vi "FTP上传UI.vi"() -> ()   [LabVIEW 2016]
uses:
  <vilib>/FTP/NI_FTP.lvlib
panel:
  out "大小（字节）":i64
  out "remote path":string
  out "temp path":path
  in  "上传版本txt":bool
  in  "read txt":bool
  in  "更新版本记录txt":string
  out "上传中":bool
  in  "remote port (21)":u16=21 caption="远程端口(21)"
  in  "password":string="std23506" caption="密码"
  in  "user":string="update" caption="用户"
  in  "host":string="27.154.58.30" caption="主机"
  in  "transfer spec":cluster{"remote path":string, "local path":path}={"remote path"="数据传输系统\\平台数据传输系统.exe\r\n", "local path"=path "C:/LabVIEW Project/builds/NEW平台数据传输系统/平台数据传输系统.exe"} caption="传输规范"
  in  "上传程序":bool
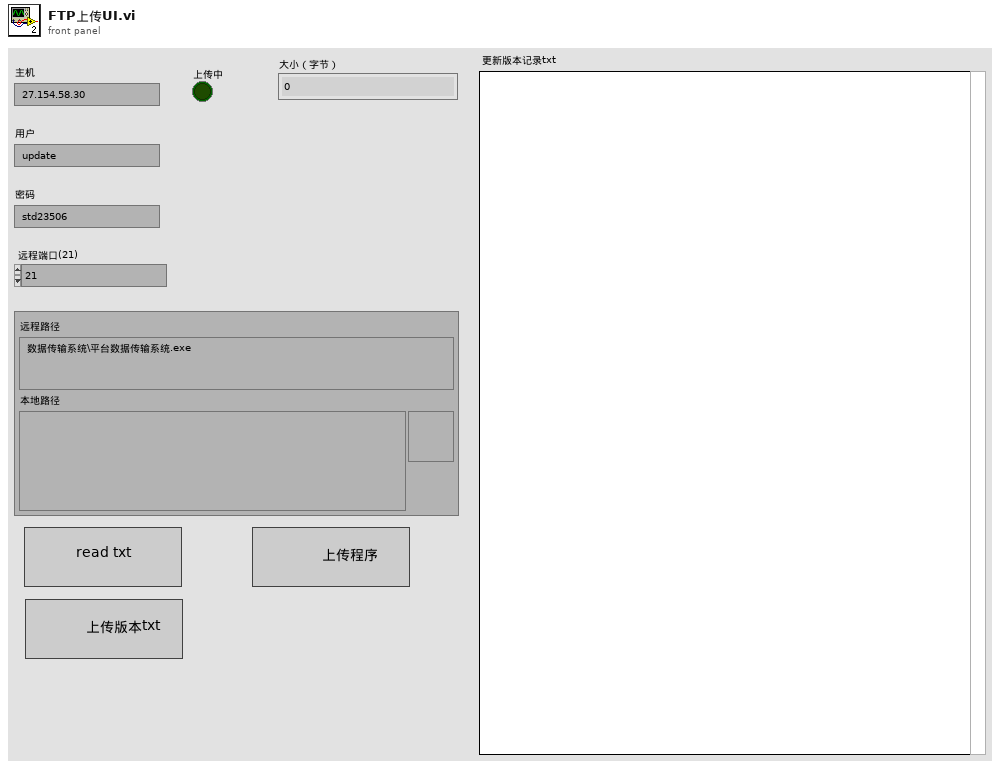
[diagram p1: front panel]
types:
  T1 = enum8{"Enabled", "Disabled", "Disabled and Grayed Out"}
  T2 = cluster{"remote path":string, "local path":path, "binary":bool}
  T3 = cluster{"remote path":string, "local path":path, "binary":bool}[]
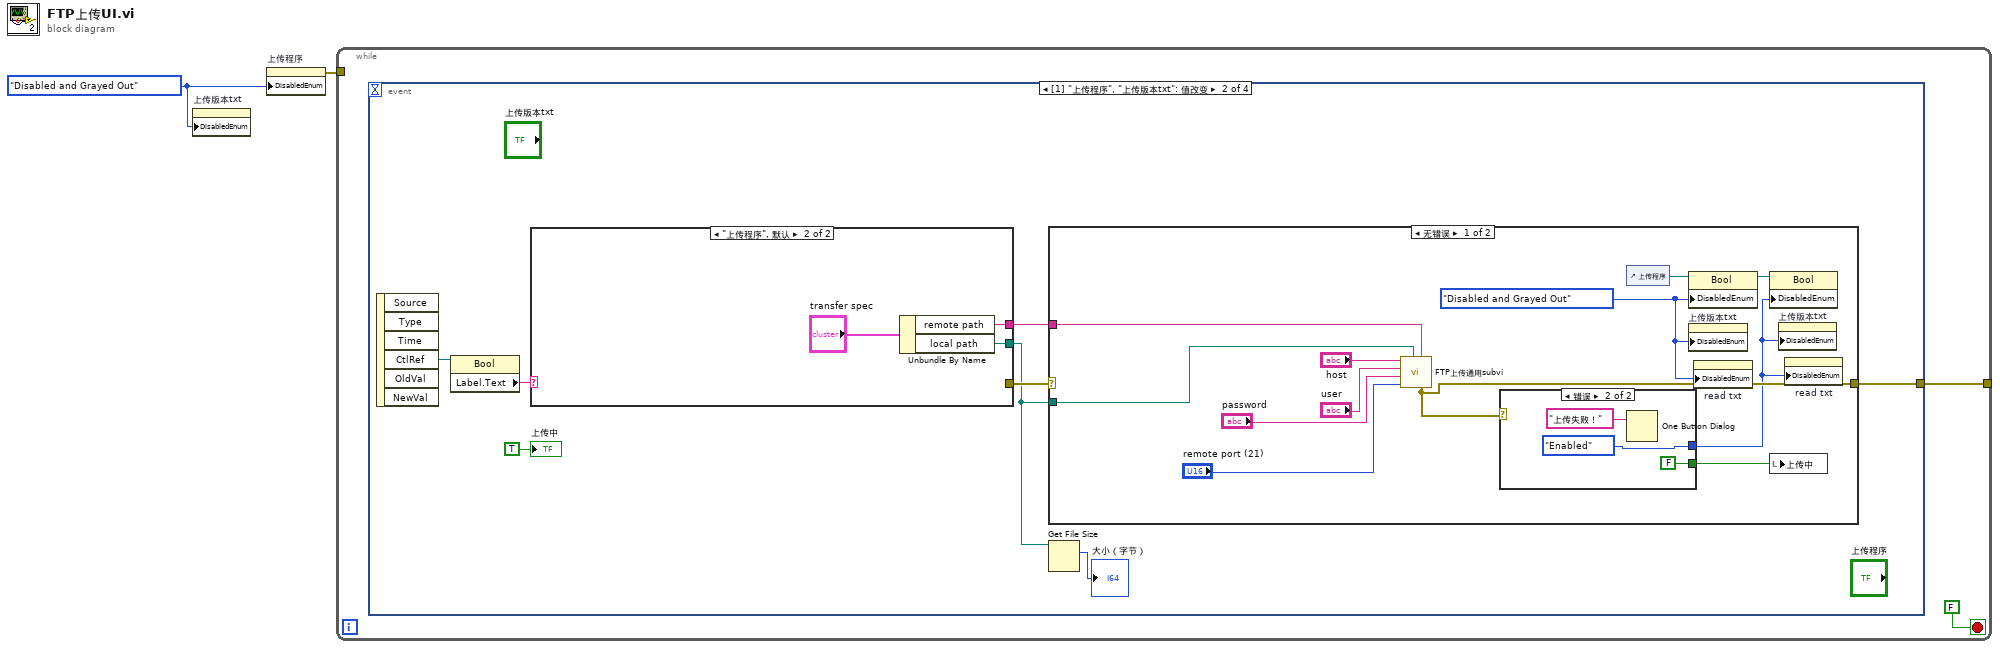
[diagram p0: block diagram]
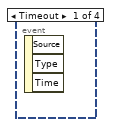
[diagram p2: hidden frame]
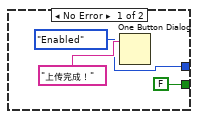
[diagram p3: hidden frame]
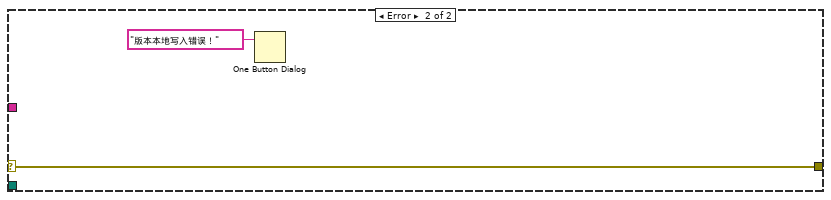
[diagram p4: hidden frame]
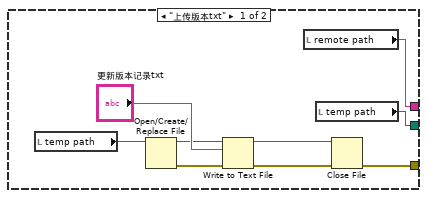
[diagram p5: hidden frame]
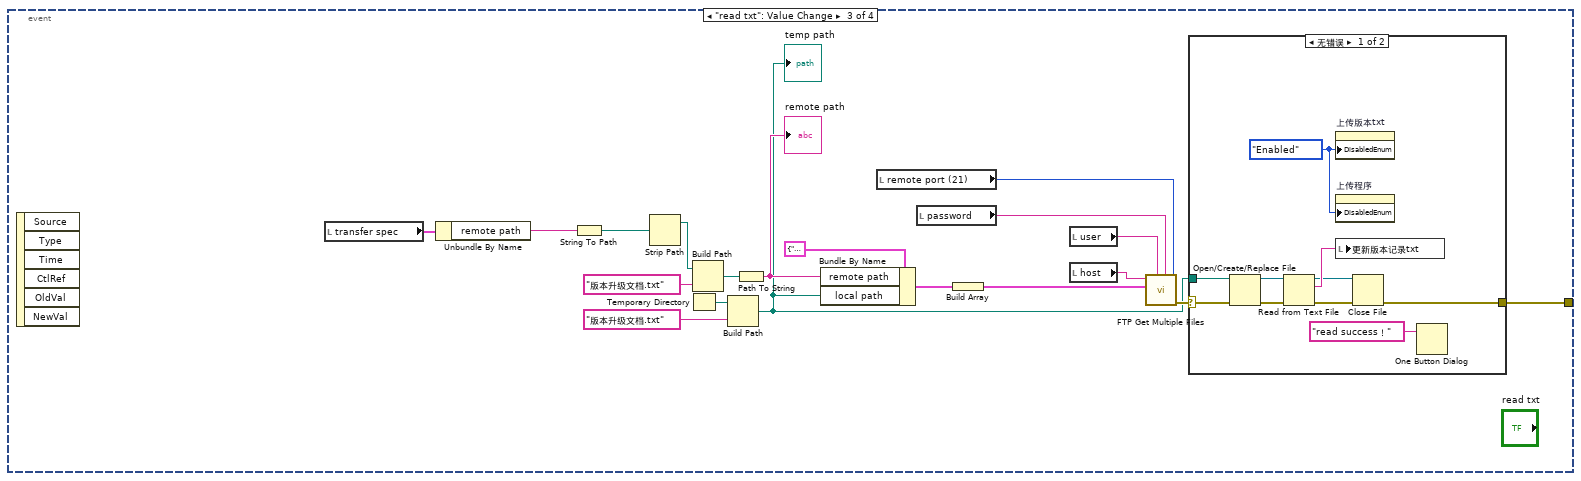
[diagram p6: hidden frame]
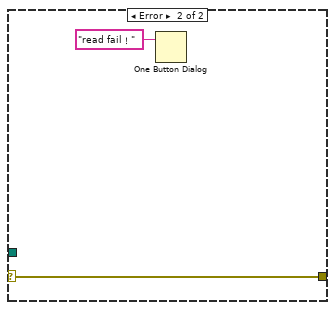
[diagram p7: hidden frame]
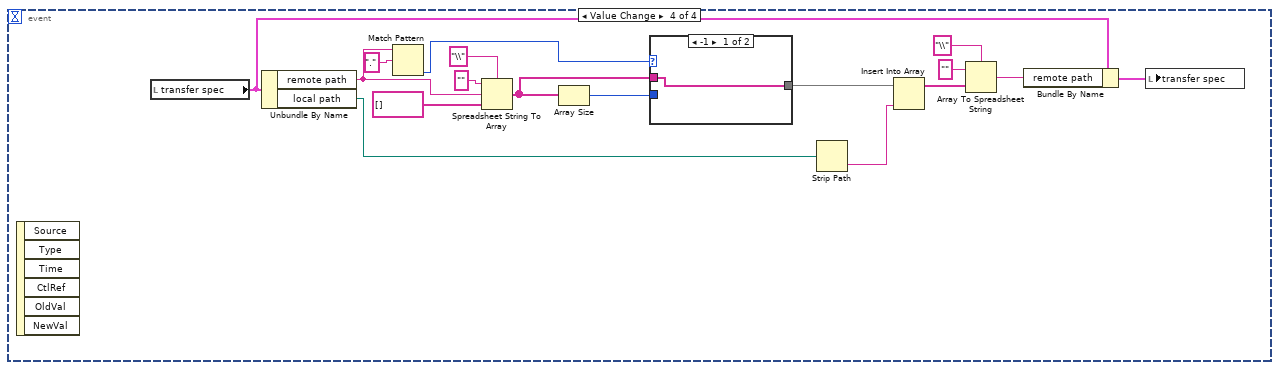
[diagram p8: hidden frame]
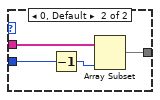
[diagram p9: hidden frame]
diagram:
  w1 = T1."Disabled and Grayed Out" ("禁用")
  n1 = property on="上传版本txt" class="Bool"("DisabledEnum"=w1) -> ()  [unwired: 2 in, 2 out]
  n2 = property on="上传程序" class="Bool"("DisabledEnum"=w1) -> (error out=w2:errorcluster)  [unwired: 2 in, 1 out]
  n3 = while {
    tunnel: [w4] -> _
    tunnel: w2 -> [_]
    stop <- FALSE stop-if-true
    n4 = event shown="[1] \"上传程序\", \"上传版本txt\": 值改变" {
      selector: _ -> [_ _ _ _]
      dyn-events: _ -> [_ _ _ _]
      timeout: _ -> [_ _ _ _]
      tunnel: [_ w12 w48 _] -> w4
      event Timeout {
        n5 = event-data() -> ()  [unwired: 1 in, 3 out]
      }
      event "上传程序", "上传版本txt": Value Change {
        n6 = event-data() -> ("CtlRef"=w10:refnum<vi>)  [unwired: 1 in, 5 out]
        n7 = property class="Bool"(reference=w10) -> ("Label.Text"=w9:string)  [unwired: 1 in, 2 out]
        n8 = case shown="\"上传程序\", 默认" w9 {
          tunnel: [w41 w43] -> w8
          tunnel: [w40 w42] -> w6
          tunnel: [w33 _] -> w7
          frame "上传版本txt" {
            n9 = local read "temp path"() -> (w39:path)
            n10 = Open/Create/Replace File(file path (use dialog)=w39) -> (refnum out=w37:refnum<file>, error out=w36:errorcluster)  [unwired: 5 in, 1 out]
            n11 = Write to Text File(file (use dialog)=w37, text="更新版本记录txt", error in=w36) -> (refnum out=w35:refnum<file>, error out=w34:errorcluster)  [unwired: 1 in, 1 out]
            n12 = local read "remote path"() -> (w41:string)
            n13 = local read "temp path"() -> (w40:path)
            n14 = Close File(refnum=w35, error in=w34) -> (error out=w33:errorcluster)  [unwired: 1 out]
          }
          frame "上传程序", Default {
            n15 = Unbundle By Name("transfer spec") -> ("remote path"=w43:string, "local path"=w42:path)
          }
        }
        n16 = case shown="无错误" w7 {
          selector: w7 -> [_ w31]
          tunnel: [w20 w31] -> w12
          tunnel: w8 -> [w16 _]
          tunnel: w6 -> [w15 _]
          frame No Error {
            w14 = T1."Disabled and Grayed Out" ("禁用")
            n17 = call "FTP上传通用subvi.vi"("remote path"=w16, "local path"=w15, "remote port (21)"="remote port (21)", "password"="password", "user"="user", "host"="host") -> ("error out"=w20:errorcluster)  [unwired: 4 in, 1 out]
            n18 = case shown="错误" w20 {
              tunnel: [FALSE FALSE] -> w19
              tunnel: [T1."Enabled" ("禁用") T1."Enabled" ("禁用")] -> w13
              frame No Error {
                n19 = One Button Dialog(message="上传完成！" ("消息")) -> ()  [unwired: 1 in, 1 out]
              }
              frame Error {
                n20 = One Button Dialog(message="上传失败！" ("消息")) -> ()  [unwired: 1 in, 1 out]
              }
            }
            n21 = control-ref of="上传程序"() -> (w18:refnum<vi>)
            n22 = property class="Bool"(reference=w18, "DisabledEnum"=w14) -> (reference out=w17:refnum<vi>)  [unwired: 1 in, 1 out]
            n23 = property on="上传版本txt" class="Bool"("DisabledEnum"=w14) -> ()  [unwired: 2 in, 2 out]
            n24 = property on="read txt" class="Bool"("DisabledEnum"=w14) -> ()  [unwired: 2 in, 2 out]
            n25 = property class="Bool"(reference=w17, "DisabledEnum"=w13) -> ()  [unwired: 1 in, 2 out]
            n26 = local write "上传中"(w19) -> ()
            n27 = property on="上传版本txt" class="Bool"("DisabledEnum"=w13) -> ()  [unwired: 2 in, 2 out]
            n28 = property on="read txt" class="Bool"("DisabledEnum"=w13) -> ()  [unwired: 2 in, 2 out]
          }
          frame Error {
            n29 = One Button Dialog(message="版本本地写入错误！" ("消息")) -> ()  [unwired: 1 in, 1 out]
          }
        }
        n30 = Get File Size(file=w6) -> (size (in bytes)=→"大小（字节）":i64)  [unwired: 1 in, 2 out]
        "上传中" <- TRUE
      }
      event "read txt": Value Change {
        n31 = event-data() -> ()  [unwired: 1 in, 6 out]
        n32 = local read "transfer spec"() -> (w58:cluster{"remote path":string, "local path":path})
        n33 = Unbundle By Name(w58) -> ("remote path"=w57:string)
        n34 = String To Path(string=w57) -> (path=w56:path)
        n35 = Strip Path(path=w56) -> (stripped path=w55:path)  [unwired: 1 out]
        n36 = Temporary Directory() -> (w46:path)
        n37 = Build Path(base path=w55, name or relative path="版本升级文档.txt" ("名称或相对路径")) -> (appended path=w53:path)
        n38 = Build Path(base path=w46, name or relative path="版本升级文档.txt" ("名称或相对路径")) -> (appended path=w45:path)
        "temp path" <- w45
        n39 = Path To String(path=w53) -> (string=w52:string)
        "remote path" <- w52
        n40 = Bundle By Name(cluster=T2 {"remote path"="", "local path"=path "", "binary"=FALSE} ("元素"), "remote path"=w52, "local path"=w45) -> (w51:T2)
        n41 = local read "remote port (21)"() -> (w60:u16)
        n42 = local read "password"() -> (w61:string)
        n43 = Build Array(w51) -> (w50:T3)
        n44 = local read "user"() -> (w62:string)
        n45 = local read "host"() -> (w63:string)
        n46 = call <vilib>:"FTP Get Multiple Files.vi"("remote port (21)"=w60, "password"=w61, "user"=w62, "file specifications"=w50, "host"=w63) -> ("error out"=w49:errorcluster)  [unwired: 5 in, 1 out]
        n47 = case shown="无错误" w49 {
          selector: w49 -> [w65 w74]
          tunnel: w45 -> [w66 _]
          tunnel: [w67 w74] -> w48
          frame No Error {
            w64 = T1."Enabled" ("禁用")
            n48 = Open/Create/Replace File(file path (use dialog)=w66, error in=w65) -> (refnum out=w71:refnum<file>, error out=w70:errorcluster)  [unwired: 4 in, 1 out]
            n49 = Read from Text File(file (use dialog)=w71, error in=w70) -> (refnum out=w69:refnum<file>, text=w73:string, error out=w68:errorcluster)  [unwired: 2 in, 1 out]
            n50 = property on="上传版本txt" class="Bool"("DisabledEnum"=w64) -> ()  [unwired: 2 in, 2 out]
            n51 = property on="上传程序" class="Bool"("DisabledEnum"=w64) -> ()  [unwired: 2 in, 2 out]
            n52 = local write "更新版本记录txt"(w73) -> ()
            n53 = Close File(refnum=w69, error in=w68) -> (error out=w67:errorcluster)  [unwired: 1 out]
            n54 = One Button Dialog(message="read success！" ("消息")) -> ()  [unwired: 1 in, 1 out]
          }
          frame Error {
            n55 = One Button Dialog(message="read fail！" ("消息")) -> ()  [unwired: 1 in, 1 out]
          }
        }
      }
      event "transfer spec.local path": Value Change {
        n56 = event-data() -> ()  [unwired: 1 in, 6 out]
        n57 = local read "transfer spec"() -> (w91:cluster{"remote path":string, "local path":path})
        n58 = Unbundle By Name(w91) -> ("remote path"=w78:string, "local path"=w92:path)
        n59 = Match Pattern(string=w78, regular expression="." ("正则表达式")) -> (offset past match=w77:i32)  [unwired: 1 in, 3 out]
        n60 = Spreadsheet String To Array(delimiter (Tab)="\\" ("分隔符(Tab)"), format string="" ("格式字符串"), spreadsheet string=w78, array type (2D Dbl)=string[] []) -> (array=w88:string[])
        n61 = Array Size(array=w88) -> (size(s)=w76:i32)
        n62 = case shown="-1" w77 {
          tunnel: w88 -> [w93 w97]
          tunnel: [w93 w96] -> w87
          tunnel: w76 -> [_ w95]
          frame -1 {
          }
          frame 0, Default {
            n63 = Decrement(x=w95) -> (x-1=w94:i32)
            n64 = Array Subset(array=w97, length=w94) -> (w96:string[])  [unwired: 1 in]
          }
        }
        n65 = Strip Path(path=w92) -> (name=w86:string)  [unwired: 1 out]
        n66 = Insert Into Array(array=w87, new element=w86) -> (w85:string[])  [unwired: 1 in]
        n67 = Array To Spreadsheet String(delimiter (Tab)="\\" ("分隔符(Tab)"), array=w85, 3:"" ("格式字符串")) -> (spreadsheet string=w84:string)
        n68 = Bundle By Name(cluster=w91, "remote path"=w84) -> (w90:cluster{"remote path":string, "local path":path})
        n69 = local write "transfer spec"(w90) -> ()
      }
    }
  }
